vi "Tinius Olsen-Loadcell.vi"() -> ()   [LabVIEW 2023]
uses:
  tinius.llb/StateM.ctl
  <vilib>/Instr/_visa.llb/VISA Configure Serial Port (Instr).vi
  <vilib>/regexp/Match Regular Expression.xnode
  <vilib>/Analysis/NI_AALBase.lvlib
panel:
  out "Force (N) 2":cluster{dbl[], dbl[]}(graph)
  out "Voltage":dbl[](array[numeric])
  in  "Zero time (s)":dbl
  out "Offset":dbl format="%0.2f"
  in  "Zero Position":bool
  in  "VISA resource name":refnum<visa-resource-name>="COM1"
  in  "Crosshead Speed [mm/s]":dbl=0.5
  in  "Zero Force":bool
  in  "Set Speed":bool
  out "saf":bool
  in  "Move Crosshead mm":dbl
  in  "Up or down":bool
  in  "?":bool
  in  "Stop":bool
  out "Displacement (mm)":dbl
  out "Elapsed Time (s)":dbl
  out "Force":dbl(graph)
  # "Tinius Olsen UI"
  # "Set controls"
  # "Measure"
  # "0mm Displacement is 1mm above the superconductor"
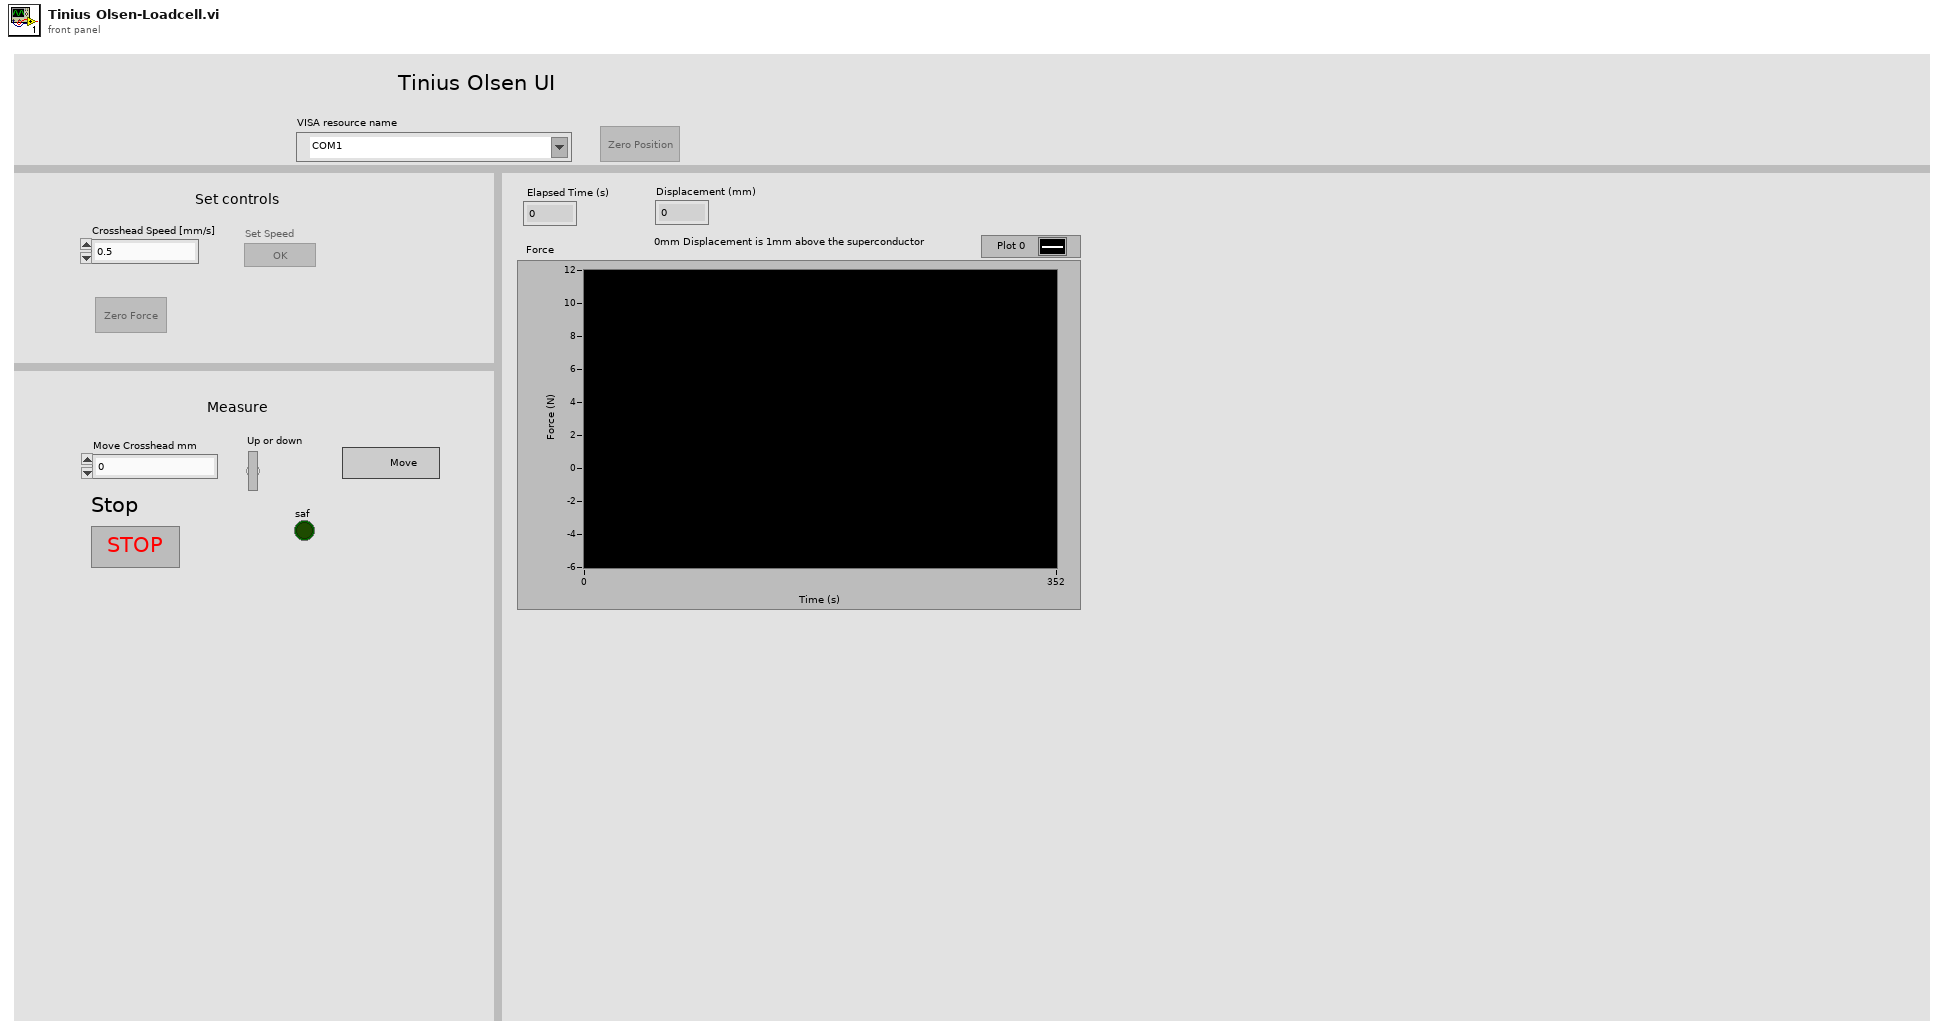
[diagram p1: front panel]
types:
  T1 = enum8{"Enabled", "Disabled", "Disabled and Grayed Out"}
  T2 = enum16{"open", "replace", "create", "open or create", "replace or create", "replace or create with confirmation"}
  T3 = typedef "StateM.ctl" = enum16{"Start", "Set controls", "Measuring", "Return", "Stop"}
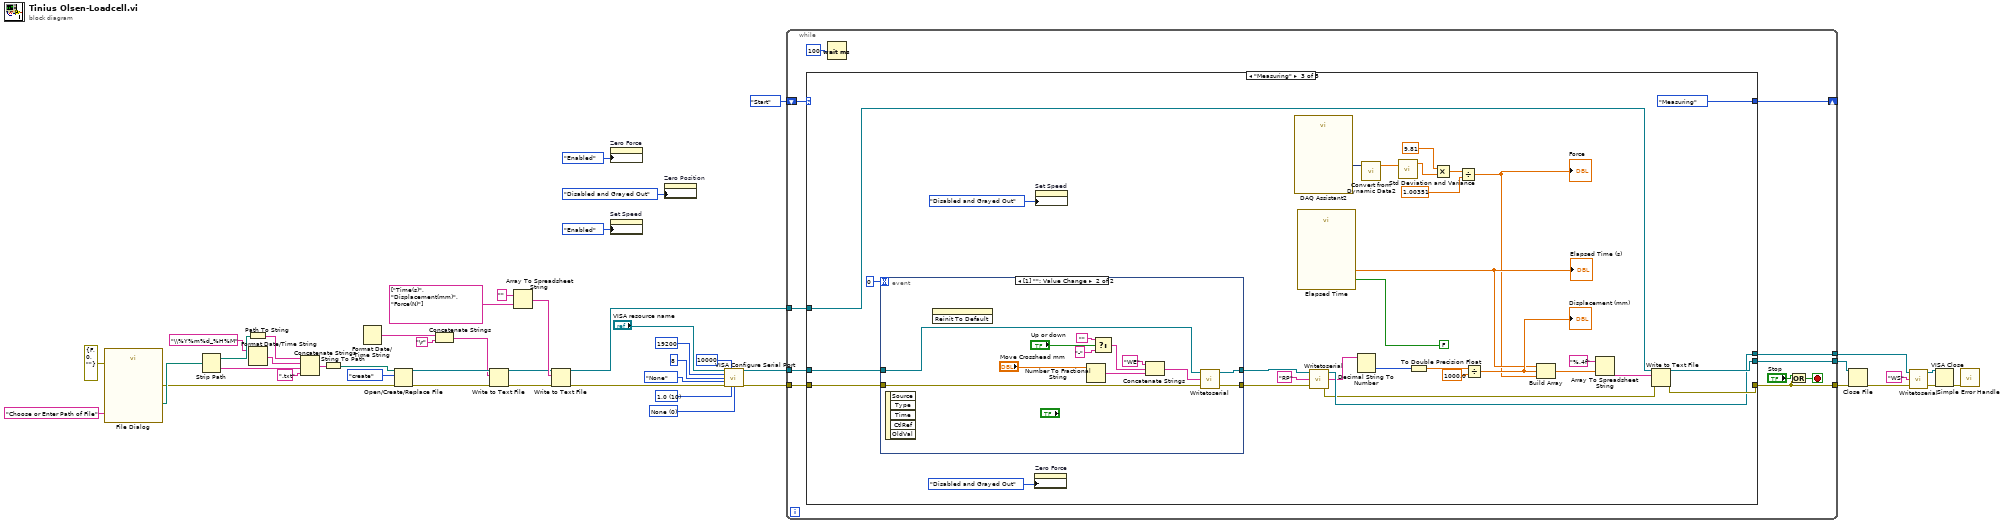
[diagram p0: block diagram]
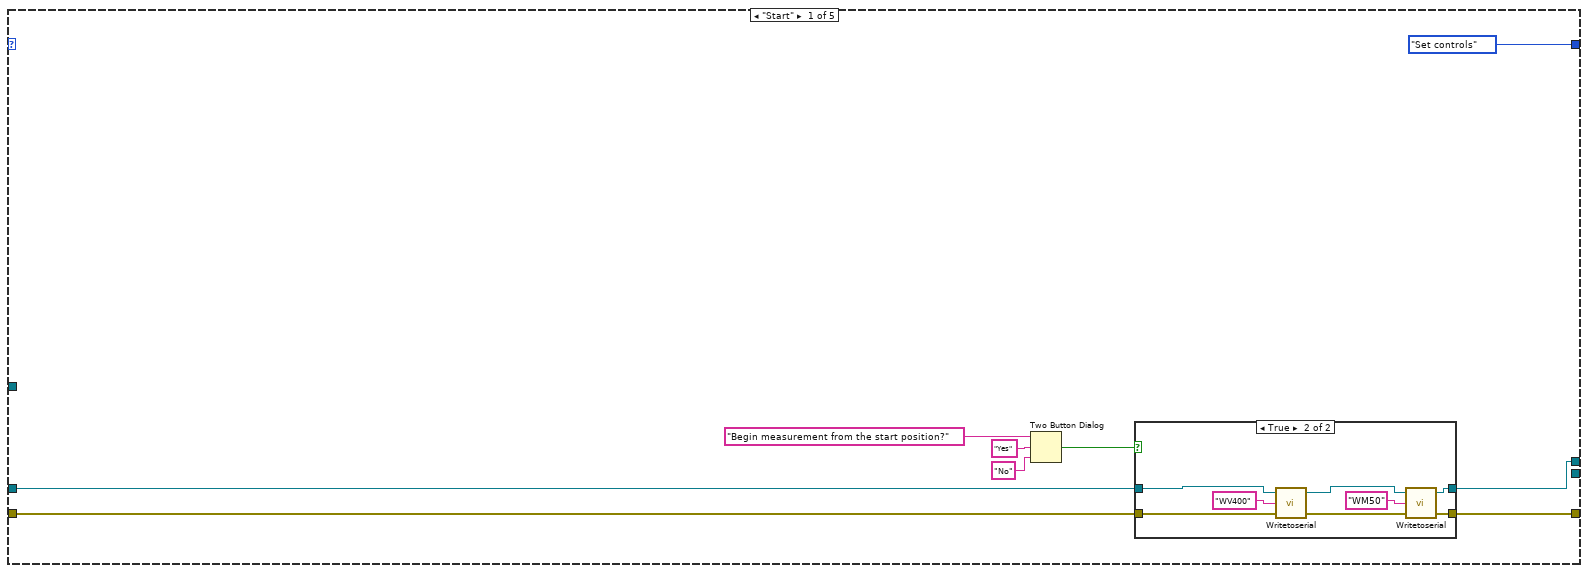
[diagram p2: hidden frame]
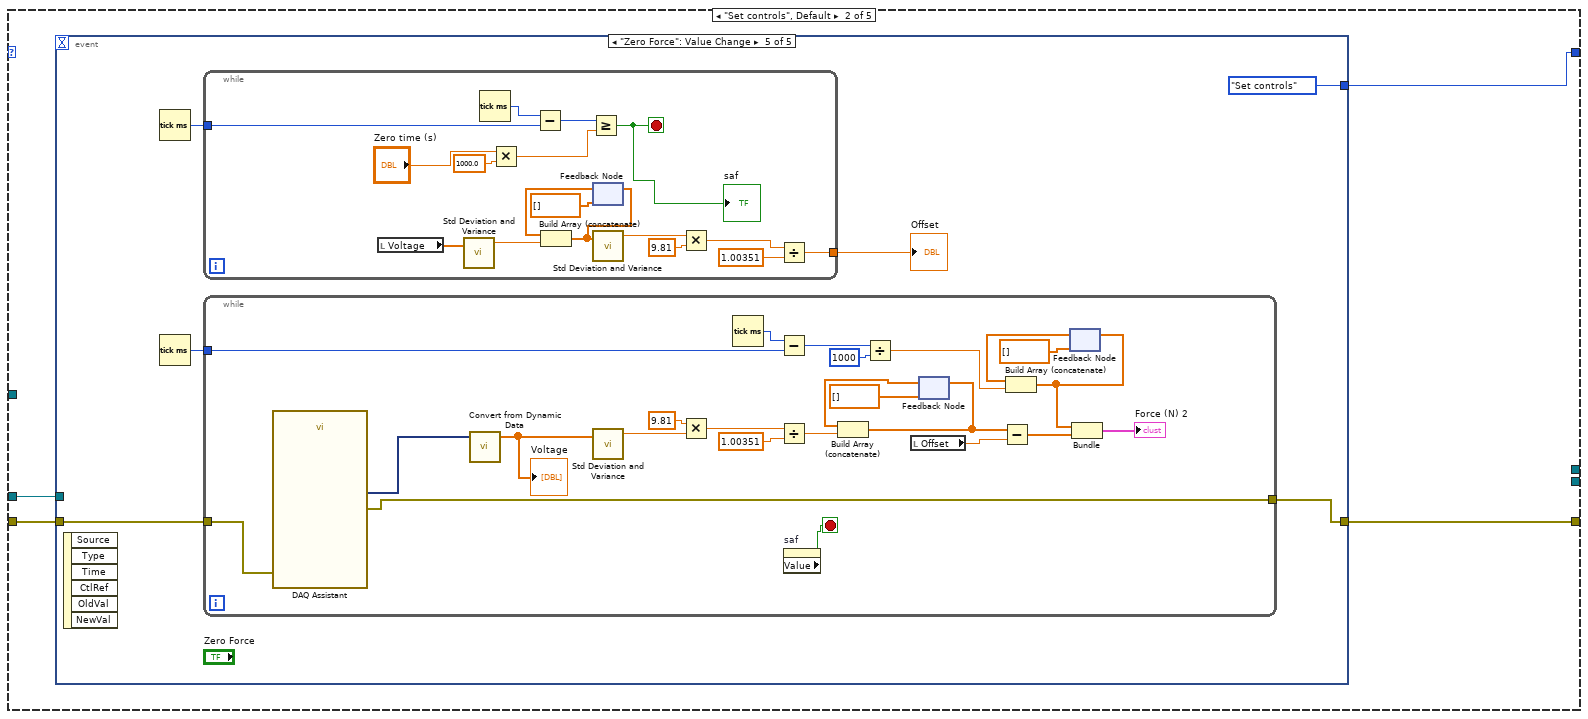
[diagram p4: hidden frame]
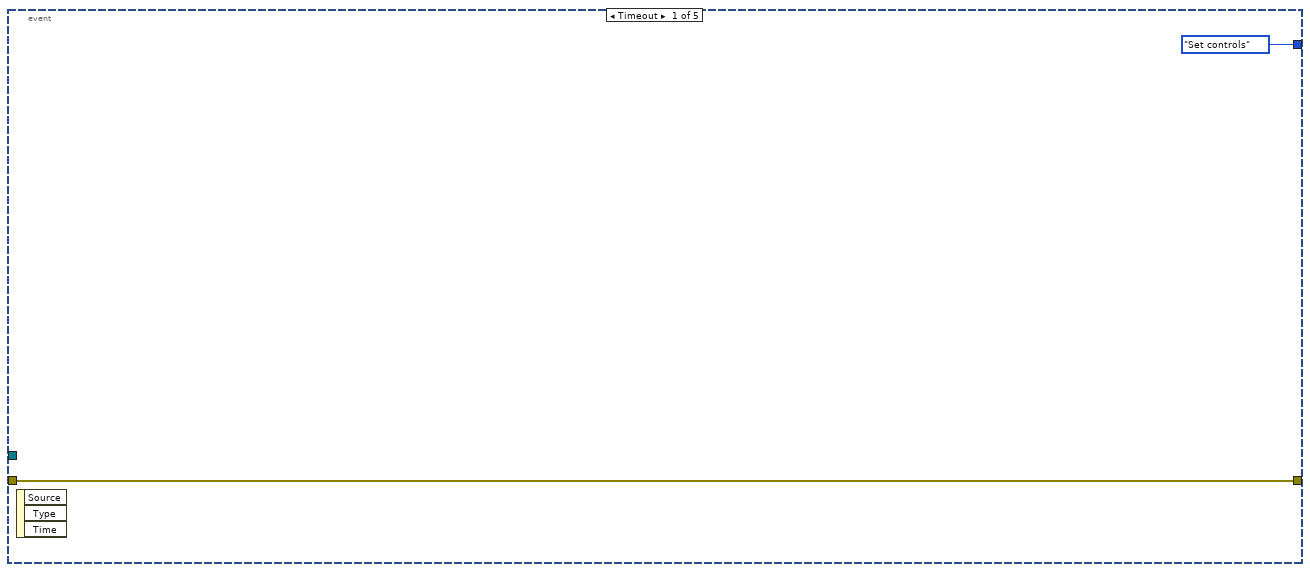
[diagram p5: hidden frame]
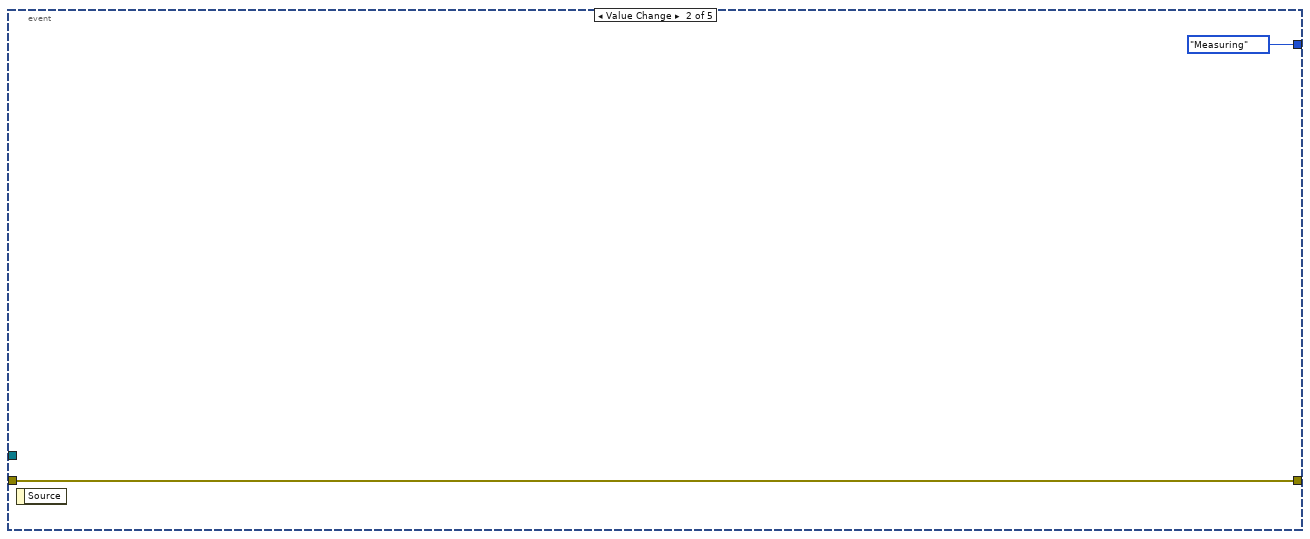
[diagram p6: hidden frame]
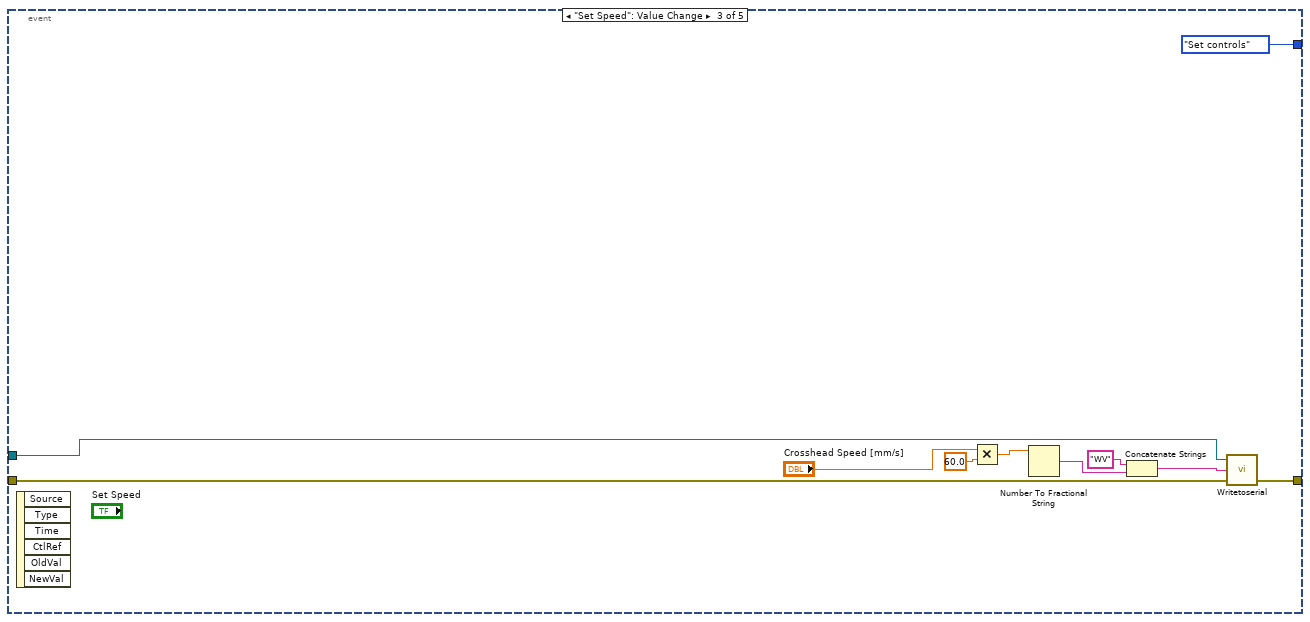
[diagram p7: hidden frame]
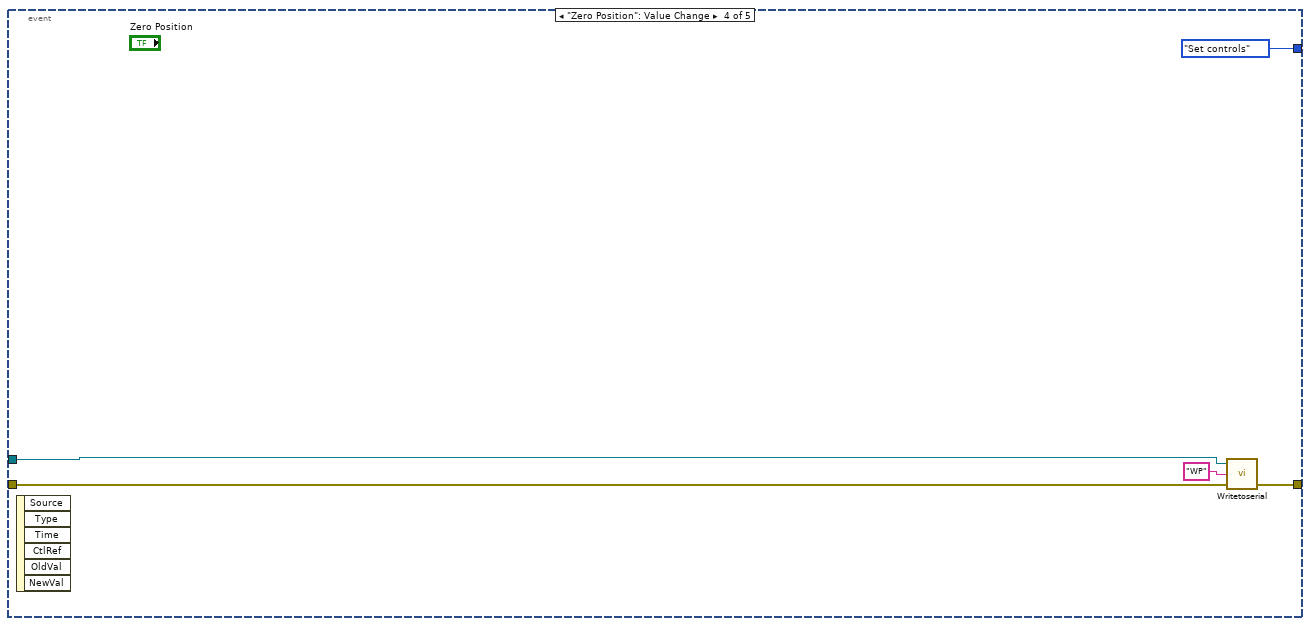
[diagram p8: hidden frame]
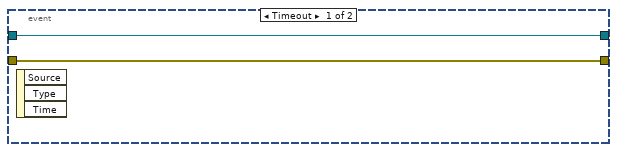
[diagram p9: hidden frame]
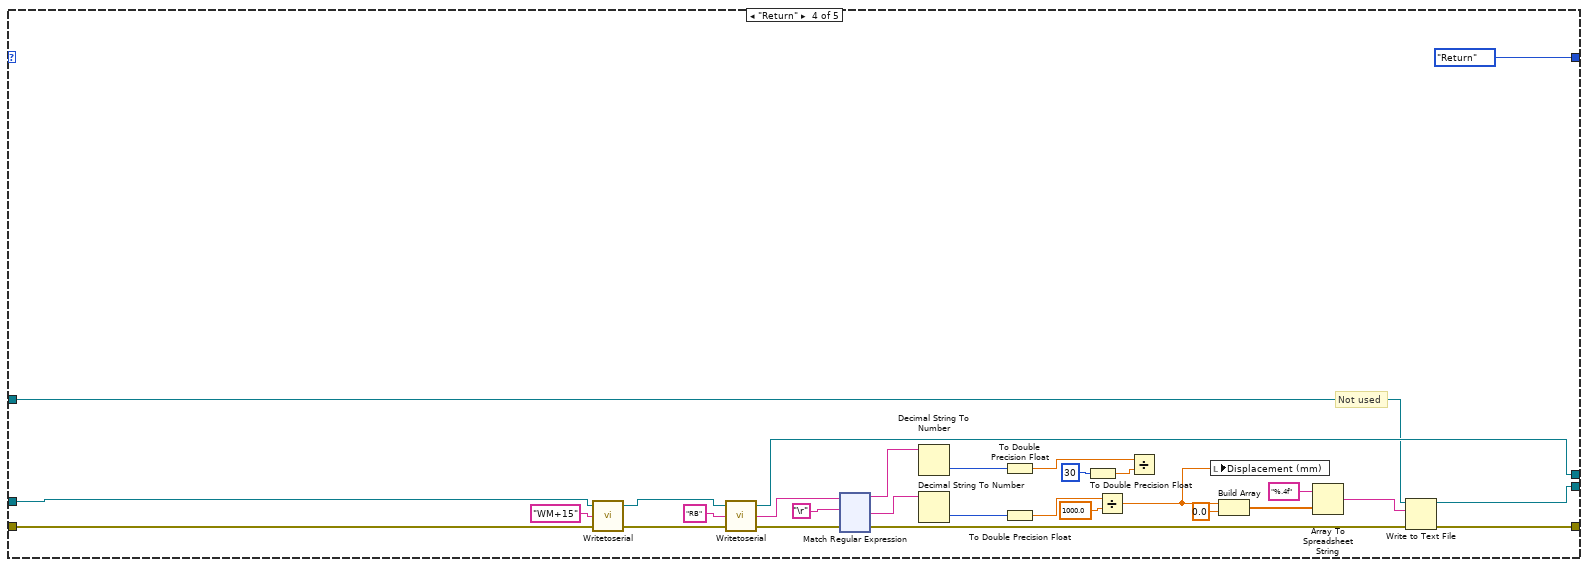
[diagram p10: hidden frame]
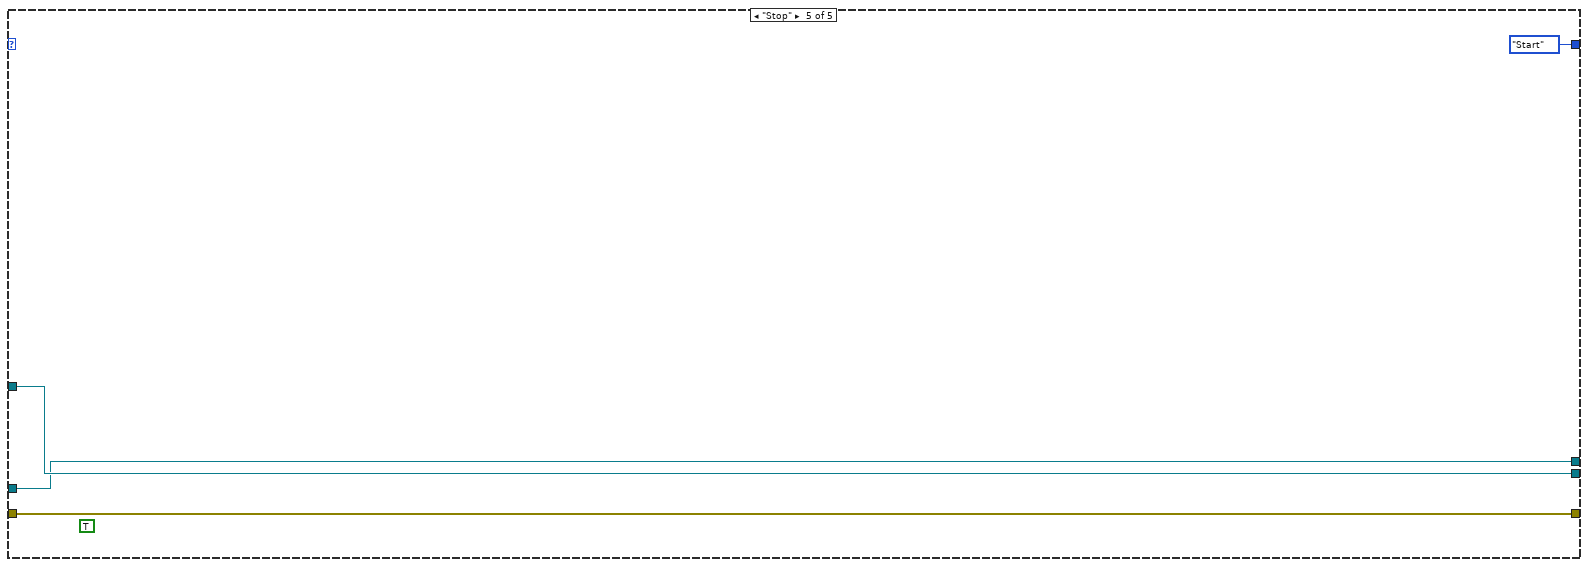
[diagram p11: hidden frame]
diagram:
  w9 = u16 0 items=["None", "XON/XOFF", "RTS/CTS", "XON/XOFF & RTS/CTS", "DTR/DSR", "XON/XOFF & DTR/DSR"] ("flow control (0:none)")
  w10 = u16 10 items=["1.0"=10, "1.5"=15, "2.0"=20] ("stop bits (10: 1 bit)")
  n1 = call "File Dialog"("prompt"="Choose or Enter Path of File", "error in"=errorcluster {"status"=FALSE, "code"=0, "source"=""} ("error constant")) -> ("selected path"=w33:path, "error out"=w24:errorcluster)  [unwired: 10 in, 2 out]
  n2 = Strip Path(path=w33) -> (stripped path=w30:path, name=w31:string)
  n3 = Path To String(path=w30) -> (string=w29:string)
  n4 = Format Date/Time String(time format string (%c)="\\%Y%m%d_%H%M" ("string")) -> (date/time string=w32:string)  [unwired: 2 in]
  n5 = Concatenate Strings(w29, w32, w31, ".txt" ("string")) -> (w28:string)
  n6 = String To Path(string=w28) -> (path=w25:path)
  n7 = Format Date/Time String() -> (date/time string=w38:string)  [unwired: 3 in]
  n8 = Open/Create/Replace File(file path (use dialog)=w25, error in=w24, operation (0:open)=T2."create") -> (refnum out=w42:refnum<file>, error out=w39:errorcluster)  [unwired: 3 in, 1 out]
  n9 = Concatenate Strings(w38, "\r") -> (w36:string)
  n10 = Write to Text File(file (use dialog)=w42, text=w36, error in=w39) -> (refnum out=w41:refnum<file>, error out=w40:errorcluster)  [unwired: 1 in, 1 out]
  n11 = Array To Spreadsheet String(array=string[] ["Time(s)", "Displacement(mm)", "Force(N)"], 3:"") -> (spreadsheet string=w46:string)  [unwired: 1 in]
  n12 = Write to Text File(file (use dialog)=w41, text=w46, error in=w40) -> (refnum out=w19:refnum<file>, error out=w20:errorcluster)  [unwired: 1 in, 1 out]
  n13 = property on="Zero Force" class="Bool (strict)"("DisabledEnum"=T1."Enabled" ("Disabled")) -> ()  [unwired: 2 in, 2 out]
  n14 = property on="Set Speed" class="Bool"("DisabledEnum"=T1."Enabled" ("Disabled")) -> ()  [unwired: 2 in, 2 out]
  n15 = property on="Zero Position" class="Bool (strict)"("DisabledEnum"=T1."Disabled and Grayed Out" ("Disabled")) -> ()  [unwired: 2 in, 2 out]
  n16 = call-poly "VISA Configure Serial Port"("VISA resource name"="VISA resource name", "timeout (10sec)"=u32 10000, "baud rate (9600)"=u32 19200, "data bits (8)"=u16 8, "parity (0:none)"=enum16{"None", "Odd", "Even", "Mark", "Space"}."None", "error in (no error)"=w20, "stop bits (10: 1 bit)"=w10, "flow control (0:none)"=w9) -> ("VISA resource name out"=w15:refnum<visa-resource-name>, "error out"=w14:errorcluster)  [unwired: 6 in]
  n17 = while {
    shift-right: [w54] -> _
    shift-left: StateM."Start" -> [w57]
    tunnel: w15 -> [w56]
    tunnel: w14 -> [w55]
    tunnel: w19 -> [w53]
    tunnel: [w47] -> w18
    tunnel: [w52] -> w17
    tunnel: [w50] -> w8
    stop <- w51 stop-if-true
    n18 = case shown="\"Measuring\"" w57 {
      tunnel: w56 -> [w63 w80 w162 w199 w339]
      tunnel: w55 -> [w62 w79 w161 w219 w338]
      tunnel: [StateM."Set controls" ("Enum") w77 StateM."Measuring" ("Enum") StateM."Return" ("Enum") StateM."Start" ("Enum")] -> w54
      tunnel: w53 -> [_ _ w174 w195 w340]
      tunnel: [w61 w78 w173 w196 w338] -> w47
      tunnel: [_ _ w172 w197 w340] -> w52
      tunnel: [w58 _ w166 w198 w339] -> w50
      frame "Start" {
        n19 = Two Button Dialog(message="Begin measurement from the start position?", 1:"No" ("F button name (\"Cancel\")"), 2:"Yes" ("T button name (\"OK\")")) -> (T button?=w64:bool)
        n20 = case shown="True" w64 {
          tunnel: w63 -> [w67 w70]
          tunnel: w62 -> [w68 w69]
          tunnel: [w68 w75] -> w61
          tunnel: [w67 w74] -> w58
          frame False {
          }
          frame True {
            n21 = call "Writetoserial.vi"("error out 2"=w69, "write buffer"="WV400", "VISA resource name out 2"=w70) -> ("error out"=w71:errorcluster, "VISA resource name out"=w72:refnum<visa-resource-name>)  [unwired: 1 out]
            n22 = call "Writetoserial.vi"("error out 2"=w71, "write buffer"="WM50", "VISA resource name out 2"=w72) -> ("error out"=w75:errorcluster, "VISA resource name out"=w74:refnum<visa-resource-name>)  [unwired: 1 out]
          }
        }
      }
      frame "Set controls", Default {
        n23 = event shown="[4] \"Zero Force\": Value Change" {
          selector: _ -> [_ _ _ _ _]
          dyn-events: _ -> [_ _ _ _ _]
          timeout: _ -> [_ _ _ _ _]
          tunnel: w80 -> [_ _ w85 w97 _]
          tunnel: w79 -> [w82 w83 w86 w96 w101]
          tunnel: [StateM."Set controls" ("Enum") StateM."Measuring" StateM."Set controls" ("Enum") StateM."Set controls" ("Enum") StateM."Set controls" ("Enum")] -> w77
          tunnel: [w82 w83 w87 w95 w100] -> w78
          event Timeout {
            n24 = event-data() -> ()  [unwired: 1 in, 3 out]
          }
          event Value Change {
            n25 = event-data() -> ()  [unwired: 1 in, 1 out]
          }
          event "Set Speed": Value Change {
            n26 = event-data() -> ()  [unwired: 1 in, 6 out]
            n27 = Multiply(x="Crosshead Speed [mm/s]", y=60.0) -> (x*y=w89:dbl)
            n28 = Number To Fractional String(number=w89) -> (F-format string=w92:string)  [unwired: 3 in]
            n29 = Concatenate Strings("WV", w92) -> (w93:string)
            n30 = call "Writetoserial.vi"("error out 2"=w86, "write buffer"=w93, "VISA resource name out 2"=w85) -> ("error out"=w87:errorcluster)  [unwired: 2 out]
          }
          event "Zero Position": Value Change {
            n31 = event-data() -> ()  [unwired: 1 in, 6 out]
            n32 = call "Writetoserial.vi"("error out 2"=w96, "write buffer"="WP", "VISA resource name out 2"=w97) -> ("error out"=w95:errorcluster)  [unwired: 2 out]
          }
          event "Zero Force": Value Change {
            n33 = event-data() -> ()  [unwired: 1 in, 6 out]
            n34 = Tick Count (ms)() -> (millisecond timer value=w102:u32)
            n35 = Tick Count (ms)() -> (millisecond timer value=w104:u32)
            n36 = while {
              tunnel: w102 -> [w145]
              tunnel: [w131] -> w103
              stop <- w130 stop-if-true
              n37 = local read "Voltage"() -> (w138:dbl[])
              n38 = call <vilib>:"Std Deviation and Variance.vi"("X"=w138) -> ("mean"=w137:dbl)  [unwired: 1 in, 2 out]
              n39 = Tick Count (ms)() -> (millisecond timer value=w146:u32)
              n40 = Multiply(x="Zero time (s)", y=1000.0) -> (x*y=w142:dbl)
              n41 = Subtract(x=w146, y=w145) -> (x-y=w141:u32)
              n42 = Greater Or Equal?(x=w141, y=w142) -> (x >= y?=w130:bool)
              "saf" <- w130
              n43 = feedback #1(dbl[] []) -> (w139:dbl[])
              n44 = Build Array (concatenate)(w139, w137) -> (w136:dbl[])
              n45 = feedback-in #1(w136) -> ()
              n46 = call <vilib>:"Std Deviation and Variance.vi"("X"=w136) -> ("mean"=w135:dbl)  [unwired: 1 in, 2 out]
              n47 = Multiply(x=w135, y=9.81) -> (x*y=w132:dbl)
              n48 = Divide(x=w132, y=1.00351) -> (x/y=w131:dbl)
            }
            "Offset" <- w103
            n49 = while {
              tunnel: w104 -> [w129]
              tunnel: w101 -> [w108]
              tunnel: [w107] -> w100
              stop <- w106 stop-if-true
              n50 = call "DAQ Assistant"("error in"=w108) -> ("data"=w125:dynamicdata, "error out"=w107:errorcluster)  [unwired: 15 in, 2 out]
              n51 = call "Convert from Dynamic Data"("Dynamic Data Type"=w125) -> ("Array"=w112:dbl[])  [unwired: 3 in]
              "Voltage" <- w112
              n52 = call <vilib>:"Std Deviation and Variance.vi"("X"=w112) -> ("mean"=w113:dbl)  [unwired: 1 in, 2 out]
              n53 = Multiply(x=9.81, y=w113) -> (x*y=w110:dbl)
              n54 = Tick Count (ms)() -> (millisecond timer value=w128:u32)
              n55 = Subtract(x=w128, y=w129) -> (x-y=w127:u32)
              n56 = Divide(x=w110, y=1.00351) -> (x/y=w111:dbl)
              n57 = property on="saf" class="Bool (strict)"() -> ("Value"=w106:bool)  [unwired: 2 in, 2 out]
              n58 = Divide(x=w127, y=u32 1000) -> (x/y=w121:dbl)
              n59 = local read "Offset"() -> (w117:dbl)
              n60 = feedback #2(dbl[] []) -> (w124:dbl[])
              n61 = Build Array (concatenate)(w124, w111) -> (w115:dbl[])
              n62 = feedback-in #2(w115) -> ()
              n63 = Subtract(x=w115, y=w117) -> (x-y=w116:dbl[])
              n64 = feedback #3(dbl[] []) -> (w122:dbl[])
              n65 = Build Array (concatenate)(w122, w121) -> (w119:dbl[])
              n66 = feedback-in #3(w119) -> ()
              n67 = Bundle(w119, w116) -> (→"Force (N) 2":cluster{dbl[], dbl[]})  [unwired: 1 in]
            }
          }
        }
      }
      frame "Measuring" {
        n68 = event shown="[1] \"\": Value Change" {
          selector: _ -> [_ _]
          dyn-events: _ -> [_ _]
          timeout: 0 -> [_ _]
          tunnel: w162 -> [w179 w183]
          tunnel: w161 -> [w178 w182]
          tunnel: [w178 w181] -> w160
          tunnel: [w179 w180] -> w159
          event Timeout {
            n69 = event-data() -> ()  [unwired: 1 in, 3 out]
          }
          event Value Change {
            n70 = event-data() -> ()  [unwired: 1 in, 5 out]
            n71 = invoke class="Bool (strict)" method="Reinit To Default"() -> ()  [unwired: 3 in, 3 out]
            n72 = Number To Fractional String(number="Move Crosshead mm") -> (F-format string=w188:string)  [unwired: 3 in]
            n73 = Select(t="", s="Up or down", f="-") -> (s? t:f=w187:string)
            n74 = Concatenate Strings("WE", w187, w188) -> (w189:string)
            n75 = call "Writetoserial.vi"("error out 2"=w182, "write buffer"=w189, "VISA resource name out 2"=w183) -> ("error out"=w181:errorcluster, "VISA resource name out"=w180:refnum<visa-resource-name>)  [unwired: 1 out]
          }
        }
        n76 = property on="Zero Force" class="Bool (strict)"("DisabledEnum"=T1."Disabled and Grayed Out" ("Disabled")) -> ()  [unwired: 2 in, 2 out]
        n77 = property on="Set Speed" class="Bool"("DisabledEnum"=T1."Disabled and Grayed Out" ("Disabled")) -> ()  [unwired: 2 in, 2 out]
        n78 = call "DAQ Assistant2"() -> ("data"=w153:dynamicdata)  [unwired: 16 in, 3 out]
        n79 = call "Elapsed Time"("Auto Reset"=FALSE) -> ("Elapsed Time (s)"=w165:dbl)  [unwired: 11 in, 7 out]
        "Elapsed Time (s)" <- w165
        n80 = call "Writetoserial.vi"("error out 2"=w160, "write buffer"="RP", "VISA resource name out 2"=w159) -> ("error out"=w154:errorcluster, "read buffer"=w155:string, "VISA resource name out"=w166:refnum<visa-resource-name>)
        n81 = Decimal String To Number(string=w155) -> (number=w170:i32)  [unwired: 2 in, 1 out]
        n82 = call "Convert from Dynamic Data2"("Dynamic Data Type"=w153) -> ("Array"=w150:dbl[])  [unwired: 3 in]
        n83 = call <vilib>:"Std Deviation and Variance.vi"("X"=w150) -> ("mean"=w151:dbl)  [unwired: 1 in, 2 out]
        n84 = To Double Precision Float(number=w170) -> (double precision float=w171:dbl)
        n85 = Multiply(x=9.81, y=w151) -> (x*y=w149:dbl)
        n86 = Divide(x=w149, y=1.00351) -> (x/y=w147:dbl)
        "Force" <- w147
        n87 = Divide(x=w171, y=1000.0) -> (x/y=w168:dbl)
        "Displacement (mm)" <- w168
        n88 = Build Array(w165, w168, w147) -> (w176:dbl[])
        n89 = Array To Spreadsheet String(array=w176, 3:"%.4f" ("format string")) -> (spreadsheet string=w175:string)  [unwired: 1 in]
        n90 = Write to Text File(file (use dialog)=w174, text=w175, error in=w154) -> (refnum out=w172:refnum<file>, error out=w173:errorcluster)  [unwired: 1 in, 1 out]
      }
      frame "Return" {
        # "Not used"
        n91 = call "Writetoserial.vi"("error out 2"=w219, "write buffer"="WM+15", "VISA resource name out 2"=w199) -> ("error out"=w201:errorcluster, "VISA resource name out"=w200:refnum<visa-resource-name>)  [unwired: 1 out]
        n92 = call "Writetoserial.vi"("error out 2"=w201, "write buffer"="RB", "VISA resource name out 2"=w200) -> ("error out"=w204:errorcluster, "read buffer"=w205:string, "VISA resource name out"=w198:refnum<visa-resource-name>)
        n93 = xnode "Match Regular Expression"("input string"=w205, "regular expression"="\r", "error in"=w204) -> ("before match"=w214:string, "after match"=w209:string, "error out"=w202:errorcluster)  [unwired: 3 in, 2 out]
        n94 = Decimal String To Number(string=w214) -> (number=w211:i32)  [unwired: 2 in, 1 out]
        n95 = Decimal String To Number(string=w209) -> (number=w207:i32)  [unwired: 2 in, 1 out]
        n96 = To Double Precision Float(number=w211) -> (double precision float=w210:dbl)
        n97 = To Double Precision Float(number=w207) -> (double precision float=w208:dbl)
        n98 = To Double Precision Float(number=30 ("Counts per full scale")) -> (double precision float=w212:dbl)
        n99 = Divide(x=w208, y=1000.0) -> (x/y=w193:dbl)
        n100 = Divide(x=w210, y=w212) -> ()  [unwired: 1 out]
        n101 = local write "Displacement (mm)"(w193) -> ()
        n102 = Build Array(w193, 0.0 ("element")) -> (w217:dbl[])
        n103 = Array To Spreadsheet String(array=w217, 3:"%.4f" ("format string")) -> (spreadsheet string=w216:string)  [unwired: 1 in]
        n104 = Write to Text File(file (use dialog)=w195, text=w216, error in=w202) -> (refnum out=w197:refnum<file>, error out=w196:errorcluster)  [unwired: 1 in, 1 out]
      }
      frame "Stop" {
        (unwired) TRUE ("Stop")
      }
    }
    n105 = Wait (ms)(milliseconds to wait=u32 100) -> ()  [unwired: 1 out]
    n106 = Or(x="Stop", y=w47) -> (x .or. y?=w51:bool)
  }
  n107 = Close File(refnum=w17, error in=w18) -> (error out=w7:errorcluster)  [unwired: 1 out]
  n108 = call "Writetoserial.vi"("error out 2"=w7, "write buffer"="WS", "VISA resource name out 2"=w8) -> ("error out"=w6:errorcluster, "VISA resource name out"=w5:refnum<visa-resource-name>)  [unwired: 1 out]
  n109 = VISA Close(VISA resource name=w5, error in (no error)=w6) -> (error out=w16:errorcluster)
  n110 = call <vilib>:"Simple Error Handler.vi"("error in (no error)"=w16) -> ()  [unwired: 4 in, 5 out]
